vi "read_tcx_file.vi"(8 "error in":errorcluster, 11 "File Path":path) -> (0 "error out":errorcluster, 2 "Time":timestamp[](array[timestamp]), 3 "Bpm":i32[](array[numeric]))   [LabVIEW 2025]
uses:
  <vilib>/Utility/file.llb/Read Delimited Spreadsheet (string).vi
  <vilib>/regexp/Match Regular Expression.xnode
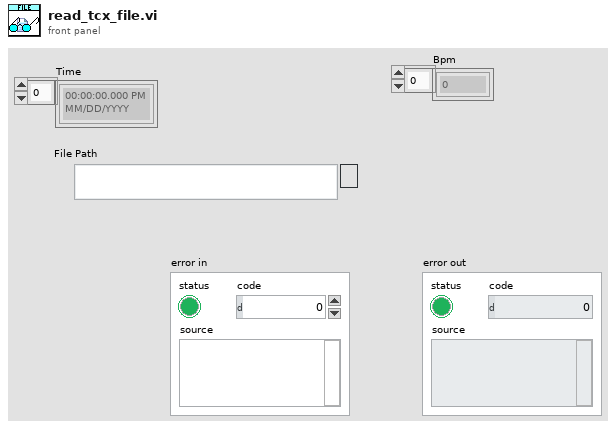
[diagram p1: front panel]
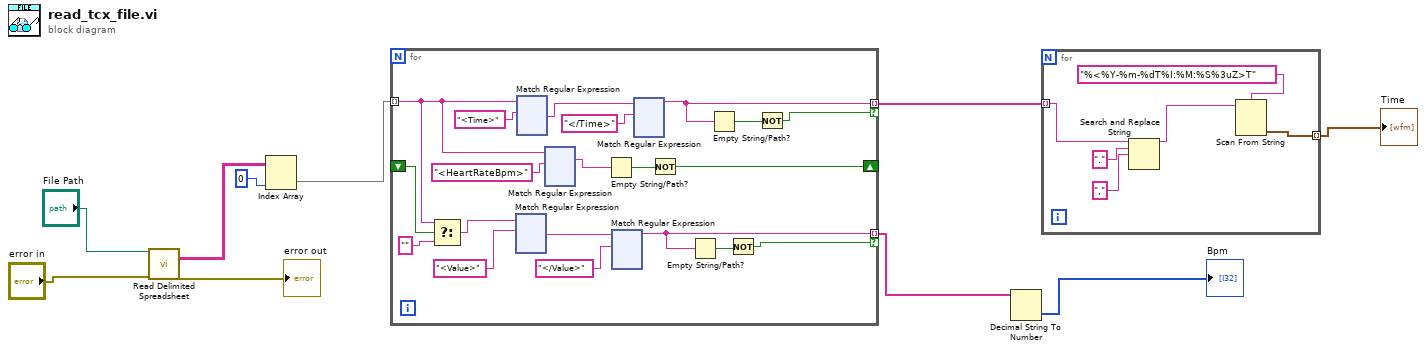
[diagram p0: block diagram]
diagram:
  n1 = call-poly <vilib>:"Read Delimited Spreadsheet.vi"("file path (dialog if empty)"="File Path", "error in (no error)"="error in") -> ("all rows"=w7:string[][], "error out"=→"error out":errorcluster)  [unwired: 8 in, 4 out]
  n2 = Index Array(array=w7, index (col)=0) -> (element=w5:string[])  [unwired: 1 in]
  n3 = for {
    tunnel: w5 -> [w22] mode=indexing
    tunnel: [w11] -> w4 mode=indexing if=w12
    shift-right: [w23] -> _
    shift-left: _ -> [w21]
    tunnel: [w14] -> w2 mode=indexing if=w13
    n4 = Select(t=w22, s=w21, f="") -> (s? t:f=w19:string)
    n5 = xnode "Match Regular Expression"("input string"=w19, "regular expression"="<Value>") -> ("after match"=w17:string)  [unwired: 4 in, 4 out]
    n6 = xnode "Match Regular Expression"("input string"=w22, "regular expression"="<Time>") -> ("after match"=w29:string)  [unwired: 4 in, 4 out]
    n7 = xnode "Match Regular Expression"("input string"=w22, "regular expression"="<HeartRateBpm>") -> ("whole match"=w25:string)  [unwired: 4 in, 4 out]
    n8 = Empty String/Path?(string/path=w25) -> (empty?=w24:bool)
    n9 = xnode "Match Regular Expression"("input string"=w17, "regular expression"="</Value>") -> ("before match"=w14:string)  [unwired: 4 in, 4 out]
    n10 = xnode "Match Regular Expression"("input string"=w29, "regular expression"="</Time>") -> ("before match"=w11:string)  [unwired: 4 in, 4 out]
    n11 = Not(x=w24) -> (.not. x?=w23:bool)
    n12 = Empty String/Path?(string/path=w14) -> (empty?=w15:bool)
    n13 = Empty String/Path?(string/path=w11) -> (empty?=w27:bool)
    n14 = Not(x=w15) -> (.not. x?=w13:bool)
    n15 = Not(x=w27) -> (.not. x?=w12:bool)
  }
  n16 = Decimal String To Number(string=w2) -> (number=→"Bpm":i32[])  [unwired: 2 in, 1 out]
  n17 = for {
    tunnel: w4 -> [w619] mode=indexing
    tunnel: [w620] -> w3 mode=indexing
    n18 = Search and Replace String(input string=w619, search string=".", replace string=",") -> (result string=w616:string)  [unwired: 5 in, 3 out]
    n19 = Scan From String(format string="%<%Y-%m-%dT%I:%M:%S%3uZ>T", input string=w616) -> (output 1=w620:timestamp)  [unwired: 3 in, 3 out]
  }
  "Time" <- w3
